vi "Dispense FN - ON - Setpoints (SubVI).vi"(0 "Main Concentration Setpoint (%)":dbl, 1 "Values IN":T1 {"Drain Time (s)" format="%.2f"; "Drain Rate (g/sec)" format="%.2f"}, 2 "Measured Mass (g)":dbl, 3 "Settings":T2={"ON Settings"={"Enable Dynamic Setpoint?"=TRUE, "Enable Dynamic Dispense Time?"=TRUE, "Enable Drain Rate Functions"=TRUE, "Dispense Sample Time (s)"=0.5, "Dispense Slope Ave"=0, "ON Timeout (sec)"=600.0, "1st Setpoint (% of Target)"=0.0, "2nd Setpoint (% of Target)"=0.0, "3rd Setpoint (% of Target)"=0.0, "Measure Dispense Delay (sec)"=0.0, "Settle Slope Sample Time (s)"=0.0}, "OFF Settings"={"Drain Sample Time (s)"=0.5, "Drain Rate Ave Size"=5, "Drain Rate Limits (± g/sec)"=10.0, "Level Slope Range (± g/sec)"=0.25, "OFF Timeout (sec)"=0.0, "Near SP Slope Level (± g/sec)"=0.01, "Near Setpoint Threshold (%)"=95.0}, "Overshoot Settings"={"Time Limit (s)"=60.0, "Container MAX (g)"=1500.0, "Max FILL Slope (+/- g/sec)"=10.0, "% Overshot to Enable (>)"=0.25}, "FILL Timeout (s)"=300.0, "Full Settle Time (s)"=3.0, "Pre-Hydrate \nSpray Time (s)"=10.0, "Pre-Hydrate \nWait Time (s)"=30.0}, 4 "State Change?":bool, 5 "Main Case Change?":bool) -> (15 "Values OUT":T1, 18 "Dynamic SP Valid?":bool, 19 "Enable Dispense Measure?":bool)   [LabVIEW 2012]
uses:
  <vilib>/ptbypt/NI_PtbyPt.lvlib
panel:
  # "Dispense Setpoints (SubVI)\nBlake Otting - October 2009"
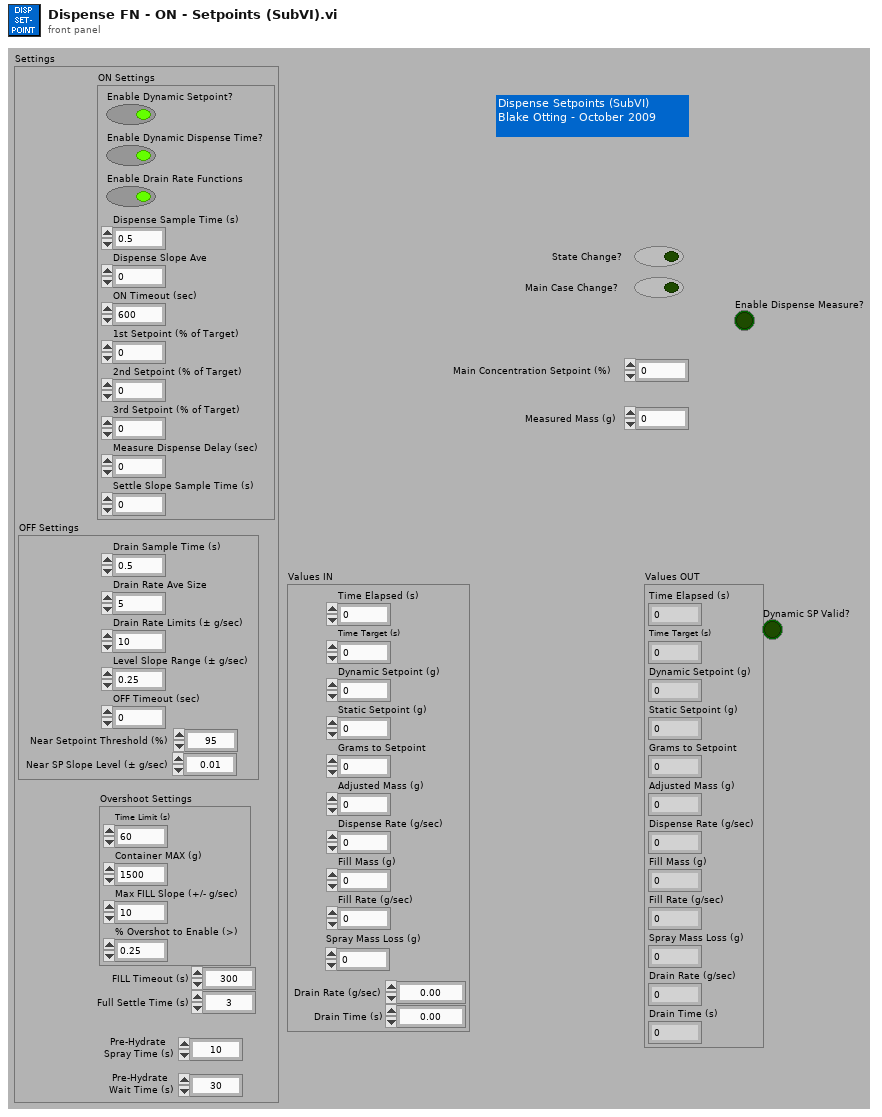
[diagram p1: front panel]
types:
  T1 = cluster{"Time Elapsed (s)":dbl, "Time Target (s)":dbl, "Dynamic Setpoint (g)":dbl, "Static Setpoint (g)":dbl, "Grams to Setpoint":dbl, "Adjusted Mass (g)":dbl, "Dispense Rate (g/sec)":dbl, "Fill Mass (g)":dbl, "Fill Rate (g/sec)":dbl, "Spray Mass Loss (g)":dbl, "Drain Rate (g/sec)":dbl, "Drain Time (s)":dbl}
  T2 = cluster{"ON Settings":cluster{"Enable Dynamic Setpoint?":bool, "Enable Dynamic Dispense Time?":bool, "Enable Drain Rate Functions":bool, "Dispense Sample Time (s)":dbl, "Dispense Slope Ave":i32, "ON Timeout (sec)":dbl, "1st Setpoint (% of Target)":dbl, "2nd Setpoint (% of Target)":dbl, "3rd Setpoint (% of Target)":dbl, "Measure Dispense Delay (sec)":dbl, "Settle Slope Sample Time (s)":dbl}, "OFF Settings":cluster{"Drain Sample Time (s)":dbl, "Drain Rate Ave Size":i32, "Drain Rate Limits (± g/sec)":dbl, "Level Slope Range (± g/sec)":dbl, "OFF Timeout (sec)":dbl, "Near SP Slope Level (± g/sec)":dbl, "Near Setpoint Threshold (%)":dbl}, "Overshoot Settings":cluster{"Time Limit (s)":dbl, "Container MAX (g)":dbl, "Max FILL Slope (+/- g/sec)":dbl, "% Overshot to Enable (>)":dbl}, "FILL Timeout (s)":dbl, "Full Settle Time (s)":dbl, "Pre-Hydrate \nSpray Time (s)":dbl, "Pre-Hydrate \nWait Time (s)":dbl}
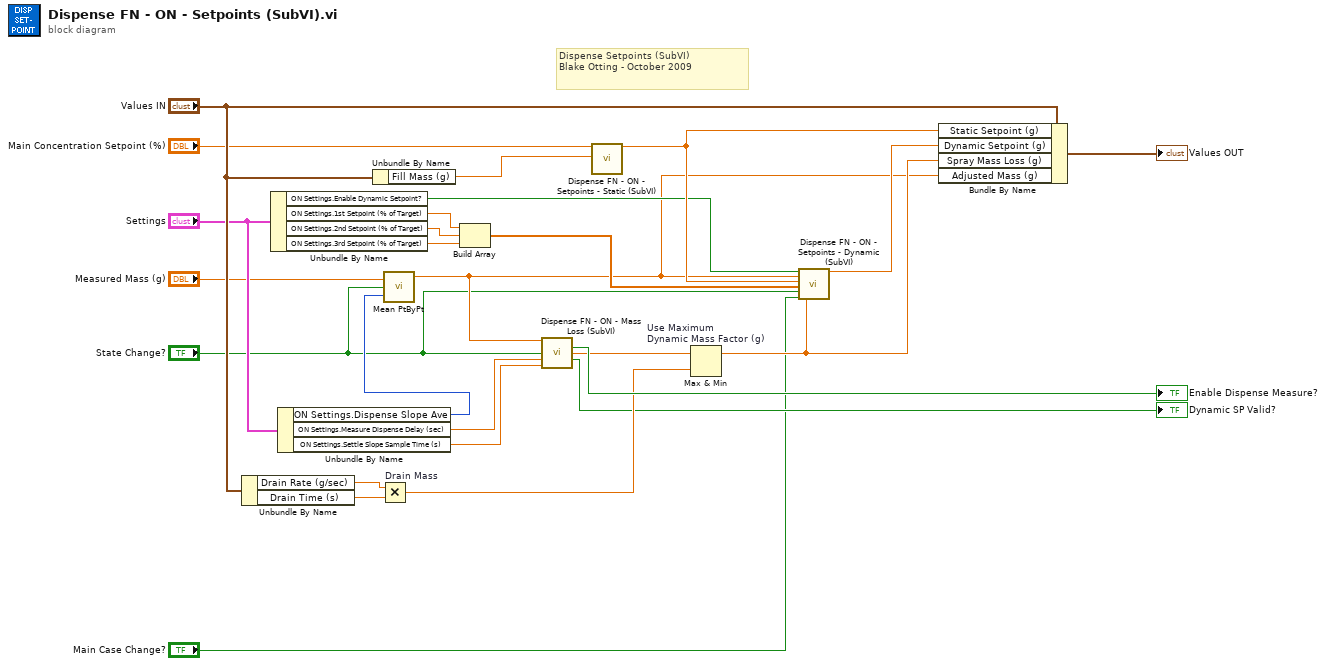
[diagram p0: block diagram]
diagram:
  # "Dispense Setpoints (SubVI)\nBlake Otting - October 2009"
  n1 = Unbundle By Name("Values IN") -> ("Drain Rate (g/sec)"=w26:dbl, "Drain Time (s)"=w25:dbl)
  n2 = Unbundle By Name("Settings") -> ("ON Settings.Enable Dynamic Setpoint?"=w11:bool, "ON Settings.1st Setpoint (% of Target)"=w17:dbl, "ON Settings.2nd Setpoint (% of Target)"=w16:dbl, "ON Settings.3rd Setpoint (% of Target)"=w15:dbl)
  n3 = Unbundle By Name("Settings") -> ("ON Settings.Dispense Slope Ave"=w6:i32, "ON Settings.Measure Dispense Delay (sec)"=w10:dbl, "ON Settings.Settle Slope Sample Time (s)"=w3:dbl)
  n4 = Unbundle By Name("Values IN") -> ("Fill Mass (g)"=w22:dbl)
  n5 = Multiply "Drain Mass"(x=w26, y=w25) -> (x*y=w13:dbl)
  n6 = call <vilib>:"Mean PtByPt.vi"("x"="Measured Mass (g)", "sample length"=w6, "initialize"="State Change?") -> ("mean"=w7:dbl)  [unwired: 2 out]
  n7 = Build Array(w17, w16, w15) -> (w14:dbl[])
  n8 = call "Dispense FN - ON - Mass Loss (SubVI).vi"("Measured Mass (g)"=w7, "State Change?"="State Change?", "Measure Dispense Delay (sec)"=w10, "Settle Slope Sample Time (s)"=w3) -> ("Enable Dispense Measure"=→"Enable Dispense Measure?":bool, "Dispense Mass Loss"=w12:dbl, "Dynamic SP Valid"=→"Dynamic SP Valid?":bool)  [unwired: 1 in, 8 out]
  n9 = call "Dispense FN - ON - Setpoints - Static (SubVI).vi"("Main Concentration Setpoint (%)"="Main Concentration Setpoint (%)", "Fill Mass (g)"=w22) -> ("Static Setpoint (g)"=w19:dbl)  [unwired: 17 out]
  n10 = Max & Min "Use Maximum\nDynamic Mass Factor (g)"(x=w12, y=w13) -> (max(x,y)=w18:dbl)  [unwired: 1 out]
  n11 = call "Dispense FN - ON - Setpoints - Dynamic (SubVI).vi"("Enable Dynamic Setpoint?"=w11, "Measured Mass (g)"=w7, "Static Setpoint (g)"=w19, "% of Setpoint per Spray"=w14, "State Change?"="State Change?", "Main Case Change?"="Main Case Change?", "Dynamic Mass Factor (g)"=w18) -> ("Dynamic Setpoint (g)"=w9:dbl)  [unwired: 6 in, 6 out]
  n12 = Bundle By Name(cluster="Values IN", "Static Setpoint (g)"=w19, "Dynamic Setpoint (g)"=w9, "Spray Mass Loss (g)"=w18, "Adjusted Mass (g)"=w7) -> (→"Values OUT":T1)
